vi "Vision V5 2-15 (vascar would be V4).vi"(0 "Image in":T2(plugin-control), 5 "error in":errorcluster) -> (14 "Histogram (Histogram 1)":u32[][](array[numeric]), 15 "Shape Report (calibrated)":T1(array[cluster]) {"Score" format="%.2f"; "Centroid"."y" format="%.2f"; "Centroid"."x" format="%.2f"}, 16 "Number of Matches":i32, 19 "error out":errorcluster)   [LabVIEW 2019]
uses:
  <vilib>/Rock Robotics/Network Tables/NT Write Number.vi
  <vilib>/Rock Robotics/Network Tables/NT Write String.vi
  <vilib>/Rock Robotics/Network Tables/NT Write Boolean.vi
  <vilib>/vision/NI_Vision_Development_Module.lvlib
panel:
  out "error out 2 (Path)":errorcluster
  in  "error in (no error) (Path)":errorcluster
  out "coerced(x)":sgl
  out "Image Out":T2(plugin-control)
  out "Histogram Graph":u32[][](graph)
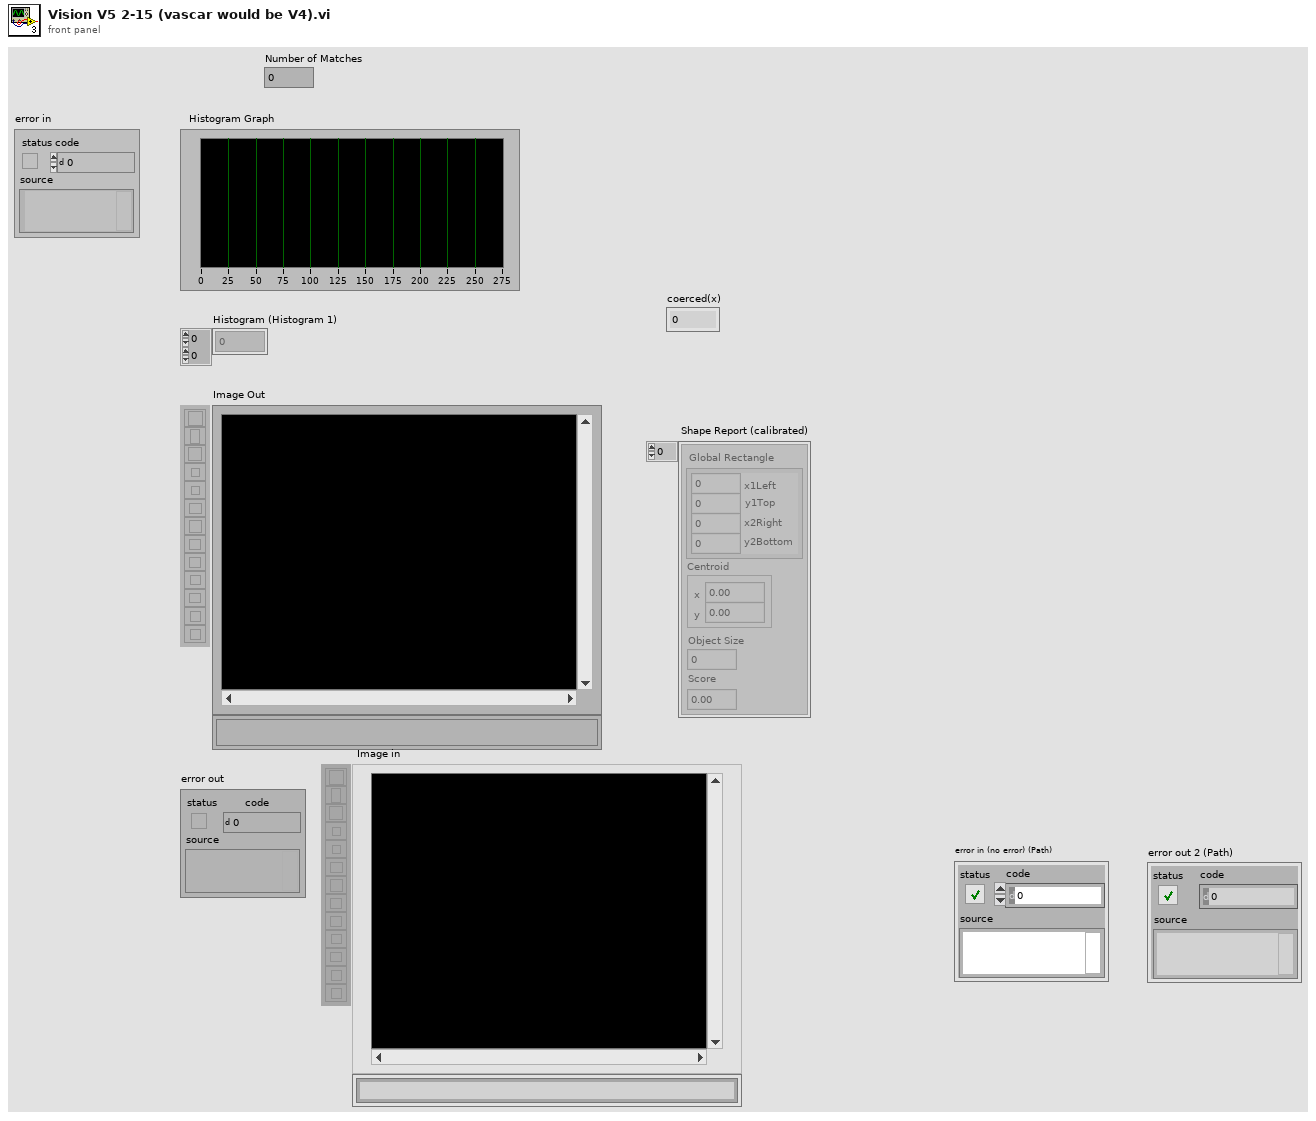
[diagram p1: front panel]
types:
  T1 = cluster{"Global Rectangle":cluster{"x1Left":i32, "y1Top":i32, "x2Right":i32, "y2Bottom":i32}, "Centroid":cluster{"x":sgl, "y":sgl}, "Object Size":u32, "Score":dbl}[]
  T2 = typedef "IMAQ Image.ctl" = refnum<image>
  T3 = cluster{"Measurement Parameter":i32, "Range Lower Value":dbl, "Range Upper Value":dbl, "Range":bool, "Measurement Type":bool}[]
  T4 = cluster{"Global Rectangle":i32[], "Contours":cluster{"ID":enum32{"External", "Internal"}, "Type":u32, "Coordinates":i32[]}[]}
  T5 = cluster{"Minimal Value":sgl, "Maximal Value":sgl, "Mean Value":sgl, "Standard  Variation":sgl, "Area (pixels)":i32}
  T6 = cluster{"histogram":u32[], "Minimal Value":sgl, "Maximal Value":sgl, "Starting Value":sgl, "Interval Width":sgl, "Mean Value":sgl, "Standard  Variation":sgl, "Area (pixels)":i32}
  T7 = typedef "Image Type" = u32
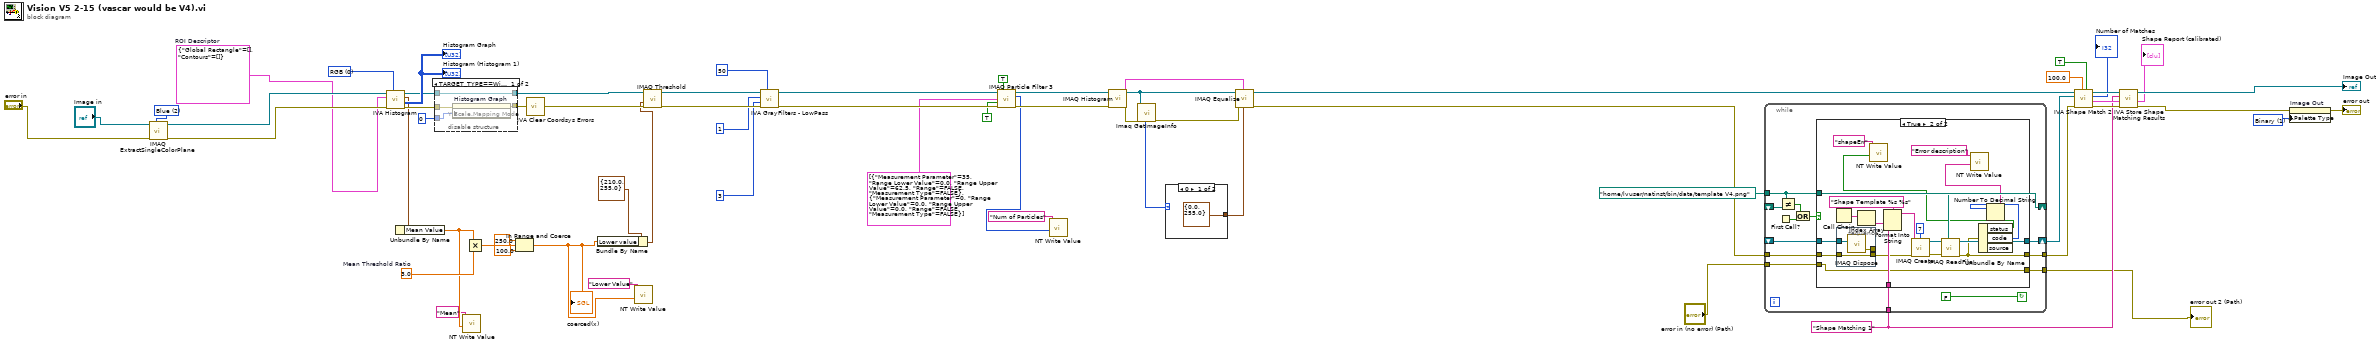
[diagram p0: block diagram]
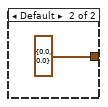
[diagram p3: hidden frame]
diagram:
  w18 = sgl 3.0  # Mean Threshold Ratio
  w20 = u32 1 items=["Grayscale", "Binary", "Gradient", "Rainbow", "Temperature", "User Defined", "Binary 16 Bit", "Gradient 16 Bit", "Rainbow 16 Bit", "Temperature 16 Bit", "User Defined 16 Bit"] ("Palette Type")
  w23 = "Shape Matching 1" ("Step Name")
  w59 = u16 0 items=["RGB", "HSL", "HSV", "HSI"] ("Color Mode")
  w57 = T4 {"Global Rectangle"=[], "Contours"=[]}  # ROI Descriptor
  w63 = 2 items=["Red", "Green", "Blue", "Hue", "Saturation", "Luminance", "Value", "Intensity"] ("Color Plane")
  n1 = call "IMAQ ExtractSingleColorPlane"("Color Plane"=w63, "error in (no error)"="error in", "Image Src"="Image in") -> ("error out"=w62:errorcluster, "Image Dst Out"=w61:T2)  [unwired: 1 in, 6 out]
  n2 = call <vilib>:"IVA Histogram.vi"("Color Mode"=w59, "error in (no error)"=w62, "ROI Descriptor"=w57, "Image In"=w61) -> ("error out"=w60:errorcluster, "Histograms"=→"Histogram Graph" →"Histogram (Histogram 1)":u32[][], "Statistics"=w19:T5, "Image Out"=w56:T2)  [unwired: 4 out]
  n3 = Unbundle By Name(w19) -> ("Mean Value"=w8:sgl)
  n4 = disable-structure "Conditional Disable Structure" shown="TARGET_TYPE==Windows" {
    disable-tunnel: w60 -> [w67 w68]
    disable-tunnel: [w66 w68] -> w54
    disable-tunnel: w56 -> [w65 w69]
    disable-tunnel: [w65 w69] -> w52
    disable-tunnel: u8 0 ("Y Scale.Mapping Mode") -> [w64 _]
    frame condition #0 {
      n5 = property on="Histogram Graph" class="WFGraph (strict)"(error in=w67, "Y Scale.Mapping Mode"=w64) -> (error out=w66:errorcluster)  [unwired: 1 in, 1 out]
    }
    frame condition #1 (active) {
    }
  }
  n6 = call-poly <vilib>:"NT Write Value.vi"("Numeric"=w8, "Name"="Mean") -> ()  [unwired: 9 in, 1 out]
  n7 = Multiply(x=w8, y=w18) -> (x*y=w16:sgl)
  n8 = In Range and Coerce(upper limit=sgl 250.0, x=w16, lower limit=sgl 100.0) -> (coerced(x)=w5:sgl)  [unwired: 1 out]
  "coerced(x)" <- w5
  n9 = call <vilib>:"IVA Clear Coordsys Errors.vi"("error in (no error)"=w54) -> ("error out"=w53:errorcluster)  [unwired: 10 in]
  n10 = Bundle By Name(cluster=cluster{"Lower value":sgl, "Upper value":sgl} {"Lower value"=210.0, "Upper value"=255.0} ("Range"), "Lower value"=w5) -> (w15:cluster{"Lower value":sgl, "Upper value":sgl})
  n11 = call-poly <vilib>:"NT Write Value.vi"("Numeric"=w5, "Name"="Lower Value") -> ()  [unwired: 9 in, 1 out]
  n12 = call "IMAQ Threshold"("error in (no error)"=w53, "Range"=w15, "Image Src"=w52) -> ("error out"=w51:errorcluster, "Image Dst Out"=w50:T2)  [unwired: 3 in, 4 out]
  n13 = call <vilib>:"IVA GrayFilters - LowPass.vi"("Tolerance"=50, "error in"=w51, "Filter size Y"=3, "Filter size X"=1, "Image In"=w50) -> ("error out"=w49:errorcluster, "Image Out"=w42:T2)  [unwired: 5 out]
  n14 = call "IMAQ Particle Filter 3"("Image Src"=w42, "Connectivity 4/8 (8)"=TRUE, "Selection Values"=T3 [{"Measurement Parameter"=35, "Range Lower Value"=0.0, "Range Upper Value"=62.5, "Range"=FALSE, "Measurement Type"=FALSE}, {"Measurement Parameter"=0, "Range Lower Value"=0.0, "Range Upper Value"=0.0, "Range"=FALSE, "Measurement Type"=FALSE}], "Keep/Remove Particles (F)"=TRUE ("Keep/Remove Particles"), "error in (no error)"=w49) -> ("Image Dst Out"=w37:T2, "Number of Particles"=w3:i32, "error out"=w43:errorcluster)  [unwired: 4 in, 4 out]
  n15 = call-poly <vilib>:"NT Write Value.vi"("Numeric"=w3, "Name"="Num of Particles") -> ()  [unwired: 9 in, 1 out]
  n16 = call "IMAQ Histogram"("error in (no error)"=w43, "Image"=w37) -> ("error out"=w36:errorcluster, "Histogram Report"=w39:T6)  [unwired: 3 in, 5 out]
  n17 = call "Imaq GetImageInfo"("error in (no error)"=w36, "Image"=w37) -> ("error out"=w35:errorcluster, "Image Type"=w38:T7)  [unwired: 8 out]
  n18 = case shown="0" w38 {
    tunnel: [cluster{"Minimum":sgl, "Maximum":sgl} {"Minimum"=0.0, "Maximum"=255.0} ("Range") cluster{"Minimum":sgl, "Maximum":sgl} {"Minimum"=0.0, "Maximum"=0.0} ("Range")] -> w34
    frame 0 {
    }
    frame Default {
    }
  }
  n19 = call "IMAQ Equalize"("Range"=w34, "Histogram Report"=w39, "error in (no error)"=w35, "Image Src"=w37) -> ("error out"=w40:errorcluster, "Image Dst Out"=w31:T2)  [unwired: 2 in, 4 out]
  n20 = while {
    shift-right: [w84] -> w24
    shift-left: _ -> [w83]
    tunnel: [w81] -> w25
    tunnel: w40 -> [w80]
    tunnel: path "/home/lvuser/natinst/bin/data/template V4.png" ("Template Path") -> [w78]
    tunnel: w23 -> [w79]
    shift-right: [w78] -> _
    shift-left: _ -> [w77]
    tunnel: [w73] -> w2
    tunnel: "error in (no error) (Path)" -> [w72]
    stop <- FALSE continue-if-true
    n21 = First Call?() -> (First Call?: T/F=w76:bool)
    n22 = Not Equal?(x=w78, y=w77) -> (x != y?=w75:bool)
    n23 = Or(x=w75, y=w76) -> (x .or. y?=w74:bool)
    n24 = case shown="True" w74 {
      tunnel: [w87 w104] -> w84
      tunnel: w83 -> [w87 w99]
      tunnel: [w86 w91] -> w81
      tunnel: w80 -> [w86 w98]
      tunnel: w78 -> [_ w92]
      tunnel: w79 -> [_ w100]
      tunnel: [w85 w96] -> w73
      tunnel: w72 -> [w85 w96]
      frame False {
      }
      frame True {
        n25 = Call Chain() -> (call chain=w102:string[])
        n26 = stacked-sequence {
          tunnel: w99 -> [w110]
          tunnel: w98 -> [w109]
          tunnel: [w109] -> w97
          tunnel: [w108] -> _
          frame #0 {
            n27 = call "IMAQ Dispose"("Image"=w110) -> ("error out"=w108:errorcluster)  [unwired: 2 in, 3 out]
          }
        }
        n28 = Index Array(array=w102) -> (element=w101:string)  [unwired: 1 in]
        n29 = Format Into String(format string="Shape Template %s %s" ("Image Name"), w101, w100) -> (resulting string=w107:string)  [unwired: 2 in, 1 out]
        n30 = call "IMAQ Create"("Border Size"=7, "Image Name"=w107, "error in (no error)"=w97) -> ("New Image"=w105:T2, "error out"=w93:errorcluster)  [unwired: 1 in, 1 out]
        n31 = call "IMAQ ReadFile"("File Path"=w92, "error in (no error)"=w93, "Image"=w105) -> ("error out"=w91:errorcluster, "Image Out"=w104:T2)  [unwired: 2 in, 5 out]
        n32 = Unbundle By Name(w91) -> ("status"=w90:bool, "code"=w89:i32)  [unwired: 1 out]
        n33 = call-poly <vilib>:"NT Write Value.vi"("Boolean"=w90, "Name"="shapeErr") -> ()  [unwired: 9 in, 1 out]
        n34 = Number To Decimal String(number=w89) -> (decimal integer string=w88:string)  [unwired: 1 in]
        n35 = call-poly <vilib>:"NT Write Value.vi"("String"=w88, "Name"="Error description") -> ()  [unwired: 9 in, 1 out]
      }
    }
  }
  "error out 2 (Path)" <- w2
  n36 = call <vilib>:"IVA Shape Match 2.vi"("Scale Invariance"=TRUE, "Minimal Score"=100.0, "error in (no error)"=w25, "Template"=w24, "Image Src"=w31) -> ("error out"=w30:errorcluster, "Shape Report"=w28:T1, "Number of Matches"=→"Number of Matches":i32, "Image Out"=w27:T2)  [unwired: 3 out]
  n37 = call <vilib>:"IVA Store Shape Matching Results.vi"("error in (no error)"=w30, "Shape Report"=w28, "Step Name"=w23, "Image in"=w27) -> ("error out"=w29:errorcluster, "Shape Report (calibrated)"=→"Shape Report (calibrated)":T1, "Image dup"=→"Image Out":T2)  [unwired: 5 out]
  n38 = property on="Image Out" class="ImageControl"(error in=w29, "Palette:Palette Type"=w20) -> (error out=→"error out":errorcluster)  [unwired: 1 in, 1 out]
